vi "ReadExecutableConfiguration.vi"(8 "Error In":errorcluster, 11 "VI Path":path) -> (0 "Error Out":errorcluster, 1 "Center On Monitor?":bool, 2 "Monitor (0 = primary)":i32, 3 "Executable Configuration":T1)   [LabVIEW 2012]
uses:
  ExecutableConfiguration.ctl
  <vilib>/Utility/config.llb/Read Key (I32).vi
  <vilib>/Utility/config.llb/Read Key (Boolean).vi
  <vilib>/Utility/config.llb/Read Key (U32).vi
  <vilib>/Utility/config.llb/Read Key (Path).vi
  libs/LV-Utilities/LV-Utilities.lvlib
  <vilib>/Utility/config.llb/NI_LVConfig.lvlib
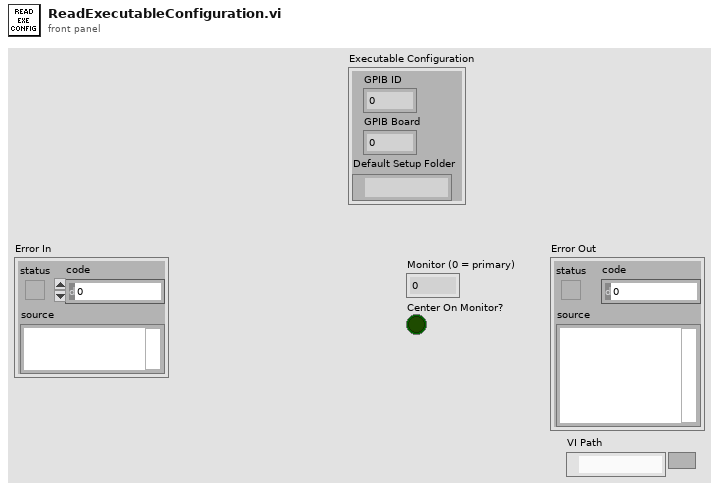
[diagram p1: front panel]
types:
  T1 = typedef "ExecutableConfiguration.ctl" = cluster{"GPIB ID":u8, "GPIB Board":u8, "Default Setup Folder":path}
  T2 = typedef "NI_LVConfig.lvlib/Config Data RefNum.ctl" = refnum<k1>
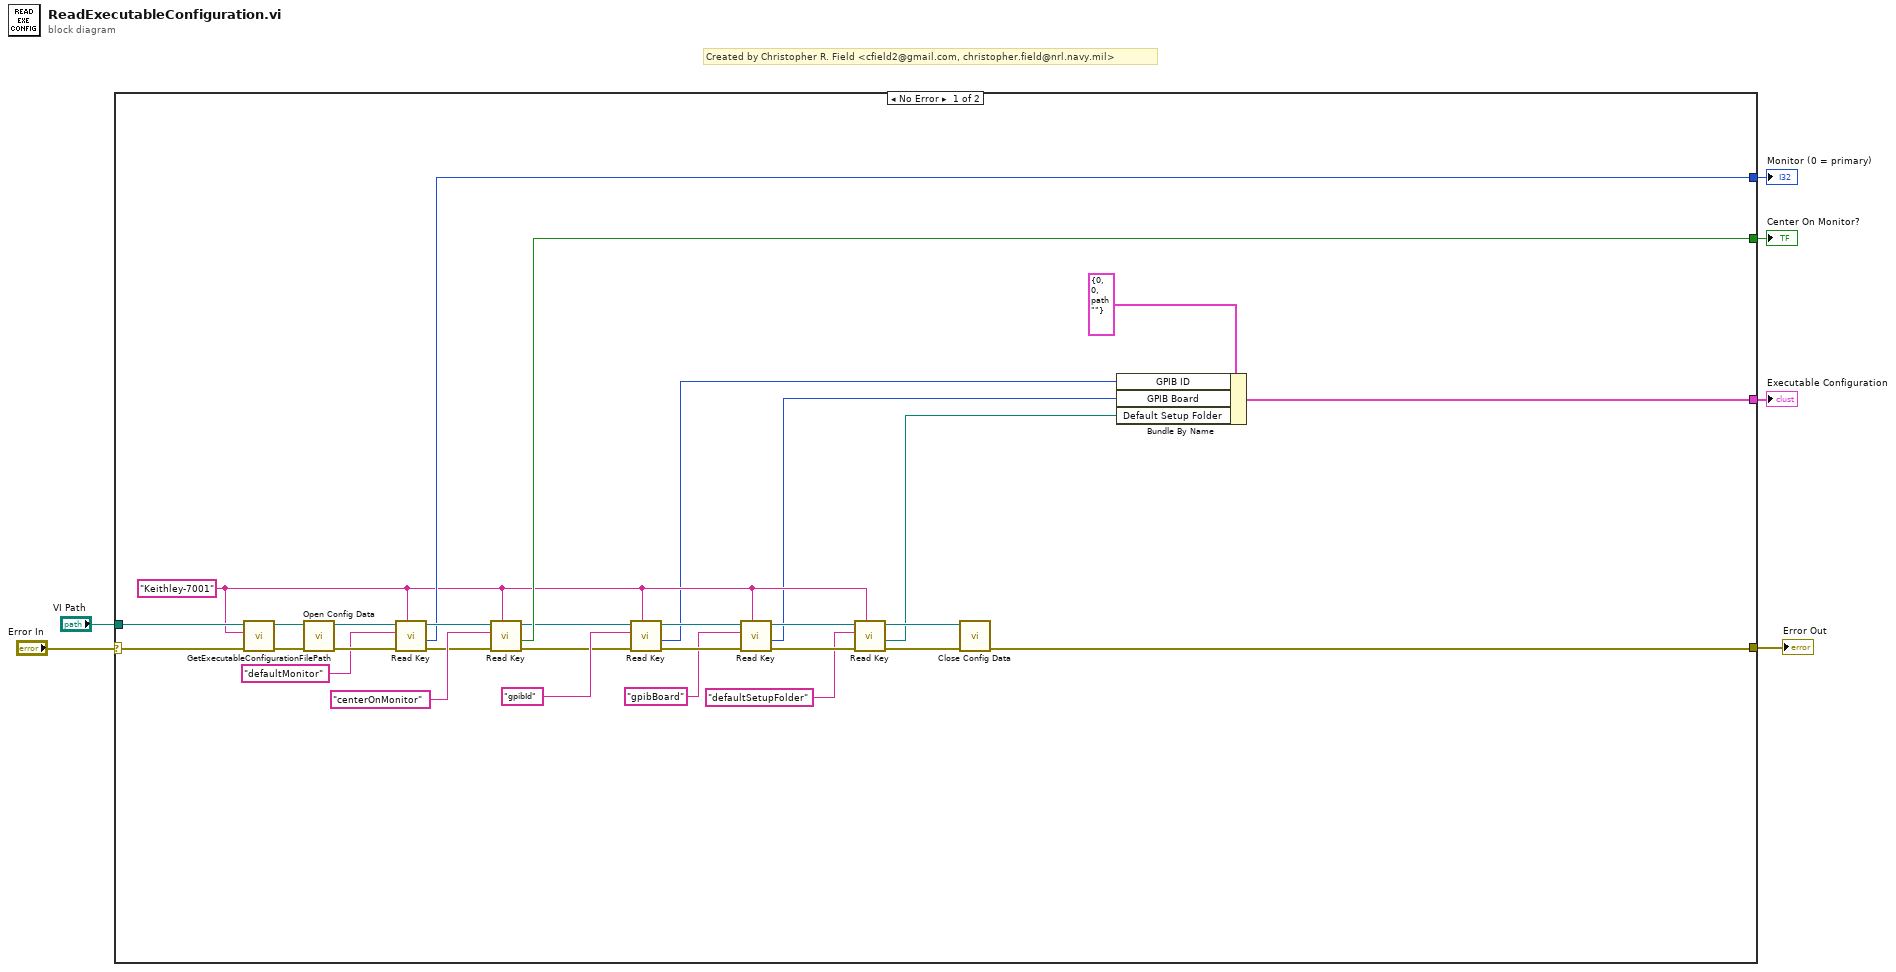
[diagram p0: block diagram]
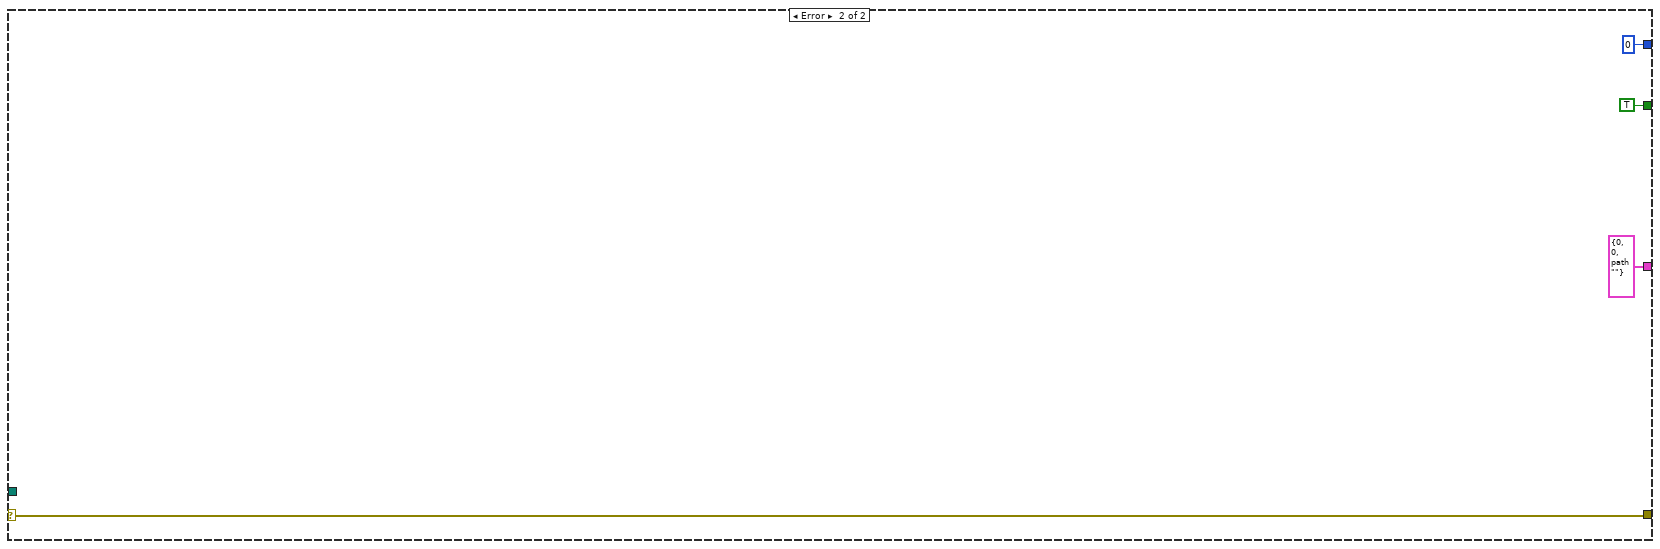
[diagram p2: hidden frame]
diagram:
  # "Created by Christopher R. Field <cfield2@gmail.com, christopher.field@nrl.navy.mil>"
  n1 = case shown="No Error" "Error In" {
    selector: "Error In" -> [w36 w40]
    tunnel: [w12 w40] -> w5
    tunnel: "VI Path" -> [w35 _]
    tunnel: [w26 0 ("value")] -> w3
    tunnel: [w25 TRUE ("value")] -> w2
    tunnel: [w7 T1 {"GPIB ID"=0, "GPIB Board"=0, "Default Setup Folder"=path ""} ("Executable Configuration")] -> w1
    frame No Error {
      w15 = "Keithley-7001" ("Application Name")
      n2 = call "GetExecutableConfigurationFilePath.vi"("Error In"=w36, "Application Name"=w15, "VI Path"=w35) -> ("Error Out"=w33:errorcluster, "Executable Config File Path"=w34:path)  [unwired: 7 in]
      n3 = call <vilib>:"Open Config Data.vi"("error in (no error)"=w33, "configuration file path"=w34) -> ("error out"=w32:errorcluster, "refnum"=w31:T2)  [unwired: 7 in, 1 out]
      n4 = call-poly <vilib>:"Read Key.vi"("section"=w15, "error in (no error)"=w32, "key"="defaultMonitor", "refnum"=w31) -> ("error out"=w28:errorcluster, "value"=w26:i32, "refnum out"=w27:T2)  [unwired: 4 in, 1 out]
      n5 = call-poly <vilib>:"Read Key.vi"("section"=w15, "error in (no error)"=w28, "key"="centerOnMonitor", "refnum"=w27) -> ("error out"=w17:errorcluster, "value"=w25:bool, "refnum out"=w19:T2)  [unwired: 4 in, 1 out]
      n6 = call-poly <vilib>:"Read Key.vi"("section"=w15, "error in (no error)"=w17, "key"="gpibId", "refnum"=w19) -> ("error out"=w23:errorcluster, "value"=w10:u32, "refnum out"=w24:T2)  [unwired: 4 in, 1 out]
      n7 = call-poly <vilib>:"Read Key.vi"("section"=w15, "error in (no error)"=w23, "key"="gpibBoard", "refnum"=w24) -> ("error out"=w20:errorcluster, "value"=w9:u32, "refnum out"=w21:T2)  [unwired: 4 in, 1 out]
      n8 = call-poly <vilib>:"Read Key.vi"("section"=w15, "error in (no error)"=w20, "key"="defaultSetupFolder", "refnum"=w21) -> ("error out"=w13:errorcluster, "value"=w8:path, "refnum out"=w14:T2)  [unwired: 4 in, 1 out]
      n9 = call <vilib>:"Close Config Data.vi"("error in (no error)"=w13, "refnum"=w14) -> ("error out"=w12:errorcluster)  [unwired: 8 in, 1 out]
      n10 = Bundle By Name(cluster=T1 {"GPIB ID"=0, "GPIB Board"=0, "Default Setup Folder"=path ""} ("Executable Configuration"), "GPIB ID"=w10, "GPIB Board"=w9, "Default Setup Folder"=w8) -> (w7:T1)
    }
    frame Error {
    }
  }
  "Error Out" <- w5
  "Monitor (0 = primary)" <- w3
  "Center On Monitor?" <- w2
  "Executable Configuration" <- w1
